vi "2D transform (DBL).vi"(6 "angle unit":u16(ring) items=["degree", "radians"], 7 "Coordenate system":cluster{"x":dbl, "y":dbl}, 8 "Scale":dbl=1.0 format="%.2f", 9 "Rotation Angle":dbl format="%.2f", 10 "Translation":cluster{"x":dbl, "y":dbl}, 11 "line endpoints":cluster{"x":dbl, "y":dbl}[](array[cluster])=[{"x"=100.0, "y"=250.0}, {"x"=90.0, "y"=250.0}, {"x"=90.0, "y"=200.0}, {"x"=95.0, "y"=175.0}, {"x"=100.0, "y"=200.0}, {"x"=100.0, "y"=250.0}]) -> (3 "tranformed line endpoint":cluster{"x":dbl, "y":dbl}[](array[cluster])=[{"x"=100.0, "y"=250.0}, {"x"=90.0, "y"=250.0}, {"x"=90.0, "y"=200.0}, {"x"=95.0, "y"=175.0}, {"x"=100.0, "y"=200.0}, {"x"=100.0, "y"=250.0}])   [LabVIEW 2017]
doc: "This VI transform (position, rotation and scale) of the a series of points from one location to another. This is used to convert points from one location to another based on \"reference\" in 2D."
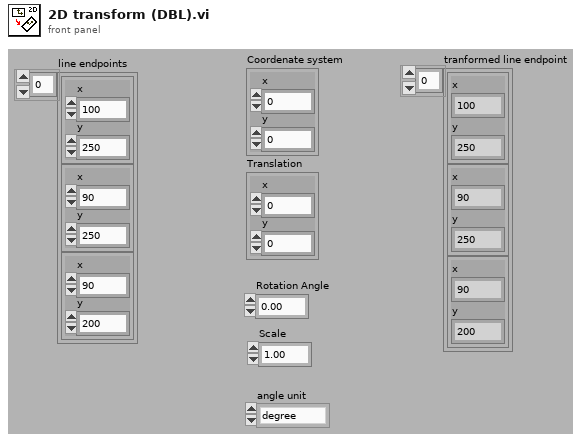
[diagram p1: front panel]
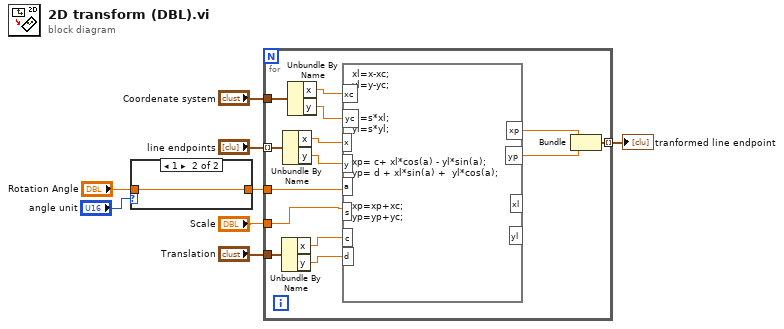
[diagram p0: block diagram]
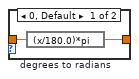
[diagram p2: hidden frame]
diagram:
  n1 = case shown="1" "angle unit" {
    tunnel: "Rotation Angle" -> [w10 w11]
    tunnel: [w9 w11] -> w2
    frame 0, Default {
      n2 = expression code="(x/180.0)*pi" "degrees to radians"(w10) -> (w9:dbl)
    }
    frame 1 {
    }
  }
  n3 = for {
    tunnel: "line endpoints" -> [w25] mode=indexing
    tunnel: "Translation" -> [w24]
    tunnel: w2 -> [w23]
    tunnel: "Scale" -> [w22]
    tunnel: [w21] -> w5 mode=indexing
    tunnel: "Coordenate system" -> [w20]
    n4 = Unbundle By Name(w24) -> ("x"=w13:dbl, "y"=w12:dbl)
    n5 = Unbundle By Name(w25) -> ("x"=w15:dbl, "y"=w14:dbl)
    n6 = Unbundle By Name(w20) -> ("x"=w17:dbl, "y"=w16:dbl)
    n7 = formula code="xl=x-xc;\nyl=y-yc;\n\n\nxl=s*xl;\nyl=s*yl;\n\n\nxp= c+ xl*cos(a) - yl*sin(a);\nyp= d + xl*sin(a) +  yl*cos(a);\n\n\nxp=xp+xc;\nyp=yp+yc;"("x"=w15, "y"=w14, "a"=w23, "s"=w22, "c"=w13, "d"=w12, "xc"=w17, "yc"=w16) -> ("xp"=w19:dbl, "yp"=w18:dbl)  [unwired: 2 out]
    n8 = Bundle("xp"=w19, "yp"=w18) -> (w21:cluster{"xp":dbl, "yp":dbl})  [unwired: 1 in]
  }
  "tranformed line endpoint" <- w5
